vi "assignment1_1.vi"() -> ()   [LabVIEW 2014]
doc: "Continuous shows the temperature values got from thermometer.vi with a waveform chart in a while loop until the user press stop button. On the panel, user can select the display of temperature scale in Celsius or Fahrenheit and summer or winter mode with different upper/lower bounds preset inside the program."
panel:
  out "minimum":dbl
  out "maximum":dbl
  out "mean":dbl
  in  "summer/winter mode":bool
  in  "Celsius/Fahrenheit":bool
  in  "stop":bool
  out "temperature analysis":T1(graph)
  out "temperature":dbl(graph)
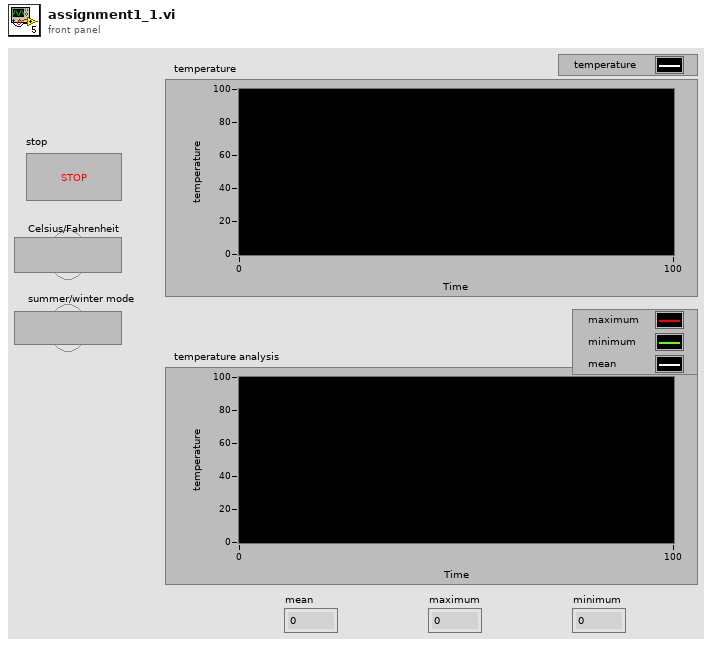
[diagram p1: front panel]
types:
  T1 = cluster{"Celsius temperature":dbl, "Celsius temperature":dbl, dbl}
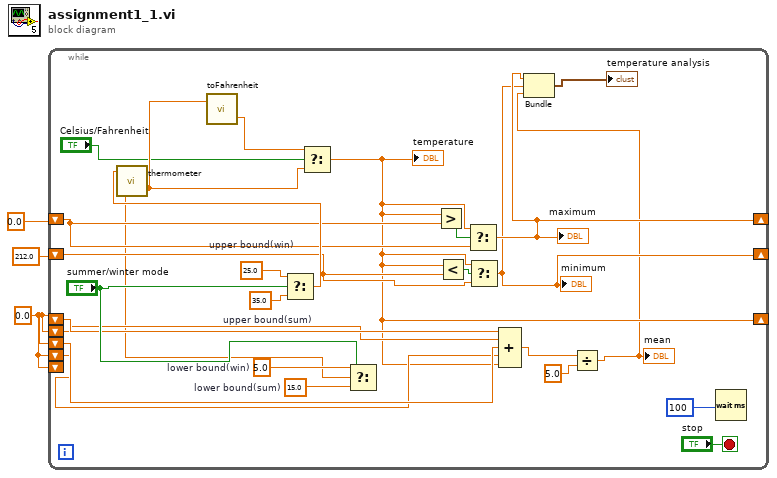
[diagram p0: block diagram]
diagram:
  w1 = 0.0
  n1 = while {
    shift-right: [w15] -> _
    shift-left: 0.0 -> [w17]
    shift-right: [w14] -> _
    shift-left: 212.0 -> [w16]
    shift-right: [w6] -> _
    shift-left: w1 -> [w10]
    shift-left: w1 -> [w9]
    shift-left: w1 -> [w8]
    shift-left: w1 -> [w7]
    shift-left: w1 -> [_]
    stop <- "stop" stop-if-true
    w24 = 5.0  # lower bound(win)
    w25 = 25.0  # upper bound(win)
    w23 = 15.0  # lower bound(sum)
    w26 = 35.0  # upper bound(sum)
    n2 = Select(t=w25, s="summer/winter mode", f=w26) -> (s? t:f=w27:dbl)
    n3 = Select(t=w24, s="summer/winter mode", f=w23) -> (s? t:f=w4:dbl)
    n4 = call "thermometer.vi"("lower  bound"=w4, "upper bound"=w27) -> ("Celsius temperature"=w30:dbl)  [unwired: 2 in]
    n5 = call "toFahrenheit.vi"("Celsius temperature"=w30) -> ("Fahrenheit temperature"=w29:dbl)  [unwired: 2 in]
    n6 = Select(t=w29, s="Celsius/Fahrenheit", f=w30) -> (s? t:f=w6:dbl)
    "temperature" <- w6
    n7 = Greater?(x=w6, y=w17) -> (0:w19:bool)
    n8 = Less?(x=w6, y=w16) -> (x < y?=w18:bool)
    n9 = Select(t=w6, s=w19, f=w17) -> (s? t:f=w15:dbl)
    "maximum" <- w15
    n10 = Select(t=w6, s=w18, f=w16) -> (s? t:f=w14:dbl)
    "minimum" <- w14
    n11 = Compound Arithmetic op=ADD(w10, w9, w8, w7, w6) -> (w11:dbl)
    n12 = Divide(x=w11, y=5.0) -> (x/y=w5:dbl)
    "mean" <- w5
    n13 = Bundle("Celsius temperature"=w15, "Celsius temperature"=w14, w5) -> (→"temperature analysis":T1)  [unwired: 1 in]
    n14 = Wait (ms)(milliseconds to wait=100) -> ()  [unwired: 1 out]
  }
